vi "List PPLs.vi"(8 "error in":errorcluster) -> (0 "error out":errorcluster, 2 "Loaded?":bool[](array[boolean]), 3 "PPL Details":T1[](array[typedef]))   [LabVIEW 2020, in "ClassLoader.lvlib"]
uses:
  ClassLoader.lvlib
  Ctl/Ctl_PPL Details.ctl
  Cache/Cache_PPL Global.vi
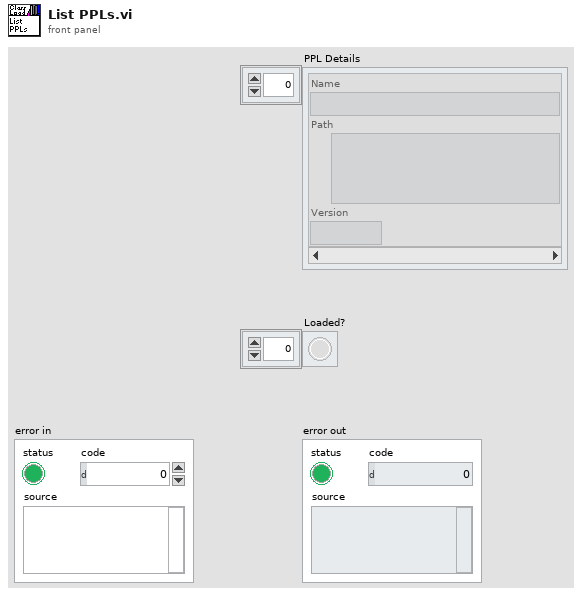
[diagram p1: front panel]
types:
  T1 = typedef "ClassLoader.lvlib/Ctl_PPL Details.ctl" = cluster{"Name":string, "Path":path, "Version":string}
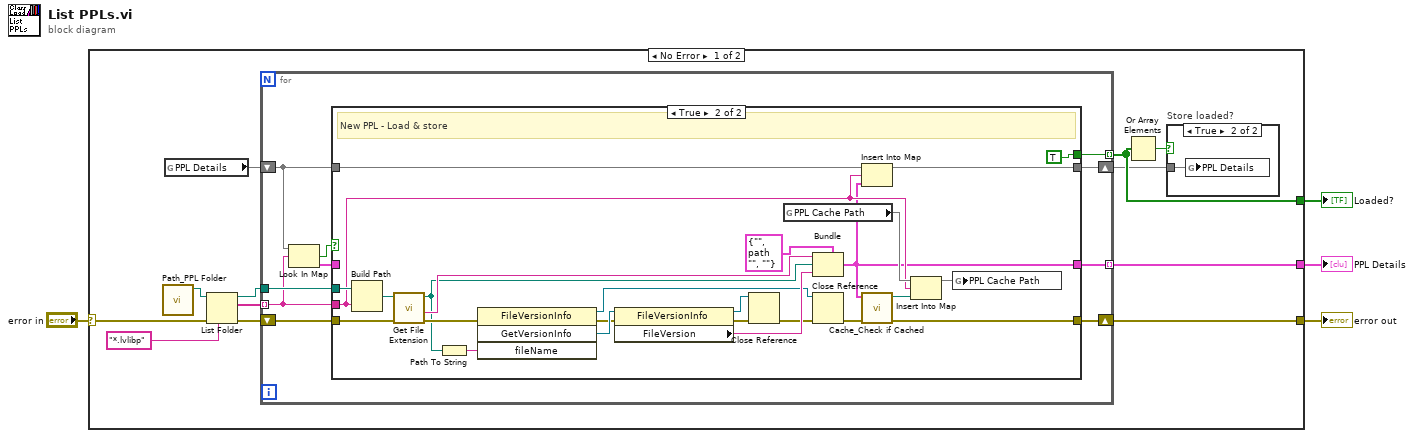
[diagram p0: block diagram]
diagram:
  n1 = case shown="No Error" "error in" {
    selector: "error in" -> [w12 w56]
    tunnel: [w10 w56] -> w3
    tunnel: [w9 _] -> w2
    tunnel: [w7 _] -> w1
    frame No Error {
      n2 = call "Path_PPL Folder.vi"() -> ("Data Folder Path"=w13:path)  [unwired: 10 in, 1 out]
      n3 = global read "Cache_PPL Global.vi" "PPL Details"() -> (w8:map{string, T1})
      n4 = List Folder(path=w13, pattern="*.lvlibp", error in=w12) -> (path out=w14:path, filenames=w15:string[], error out=w11:errorcluster)  [unwired: 1 in, 1 out]
      n5 = for {
        tunnel: w15 -> [w21] mode=indexing
        tunnel: w14 -> [w27]
        tunnel: [w24] -> w9 mode=indexing
        shift-right: [w25] -> w10
        shift-left: w11 -> [w26]
        shift-right: [w23] -> w5
        shift-left: w8 -> [w22]
        tunnel: [w18] -> w7 mode=indexing
        n6 = Look In Map(map=w22, key=w21) -> (key not found?=w20:bool, value=w19:T1)  [unwired: 1 in]
        n7 = case shown="True" w20 {
          tunnel: w27 -> [_ w54]
          tunnel: w26 -> [w29 w51]
          tunnel: [w29 w34] -> w25
          tunnel: [w30 w33] -> w24
          tunnel: [w28 w41] -> w23
          tunnel: w22 -> [w28 w39]
          tunnel: w21 -> [_ w36]
          tunnel: w19 -> [w30 _]
          tunnel: [_ TRUE] -> w18
          frame False {
            # "Key found - Return stored data"
          }
          frame True {
            # "New PPL - Load & store"
            n8 = Build Path(base path=w54, name or relative path=w36) -> (appended path=w50:path)
            n9 = call <vilib>:"Get File Extension.vi"("error in (no error)"=w51, "file"=w50) -> ("error out"=w43:errorcluster, "filename without extension"=w49:string, "dup file"=w42:path)  [unwired: 5 in, 2 out]
            n10 = Path To String(path=w42) -> (string=w53:string)
            n11 = invoke class="FileVersionInfo" method="GetVersionInfo"(error in=w43, "fileName"=w53) -> (reference out=w44:refnum<k24>, error out=w48:errorcluster, "GetVersionInfo"=w55:refnum<k24>)  [unwired: 2 in, 1 out]
            n12 = property class="FileVersionInfo"(reference=w55, error in=w48) -> (reference out=w47:refnum<k24>, error out=w46:errorcluster, "FileVersion"=w52:string)
            n13 = Close Reference(reference=w47, error in (no error)=w46) -> (error out=w45:errorcluster)
            n14 = global read "Cache_PPL Global.vi" "PPL Cache Path"() -> (w37:map{string, path})
            n15 = Bundle(cluster=T1 {"Name"="", "Path"=path "", "Version"=""}, "Name"=w49, "Path"=w42, "Version"=w52) -> (w33:T1)
            n16 = Close Reference(reference=w44, error in (no error)=w45) -> (error out=w35:errorcluster)
            n17 = Insert Into Map(map in=w39, key=w36, value=w33) -> (map out=w41:map{string, T1})  [unwired: 2 out]
            n18 = call "Cache_Check if Cached.vi"("error in"=w35, "PPL Details"=w33) -> ("error out"=w34:errorcluster, "Cache Path"=w32:path)  [unwired: 7 in, 1 out]
            n19 = Insert Into Map(map in=w37, key=w36, value=w32) -> (map out=w31:map{string, path})  [unwired: 2 out]
            n20 = global write "Cache_PPL Global.vi" "PPL Cache Path"(w31) -> ()
          }
        }
      }
      n21 = Or Array Elements(Boolean array=w7) -> (logical OR=w6:bool)
      n22 = case "Store loaded?" shown="True" w6 {
        tunnel: w5 -> [_ w17]
        frame False {
        }
        frame True {
          n23 = global write "Cache_PPL Global.vi" "PPL Details"(w17) -> ()
        }
      }
    }
    frame Error {
    }
  }
  "error out" <- w3
  "PPL Details" <- w2
  "Loaded?" <- w1
